vi "AlazarDSPGetModules.vi"(8 "error in (no error)":errorcluster, 11 "Handle":u32) -> (0 "error out":errorcluster, 1 "DSP Modules":u32[](array[numeric]), 2 "Return Code":u32, 3 "Handle":u32)   [LabVIEW 2018]
uses:
  ATSApi.dll
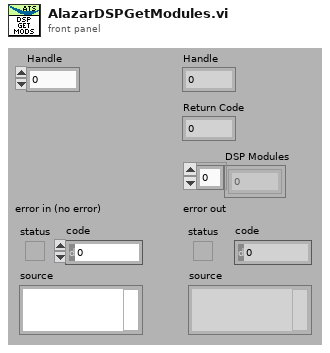
[diagram p1: front panel]
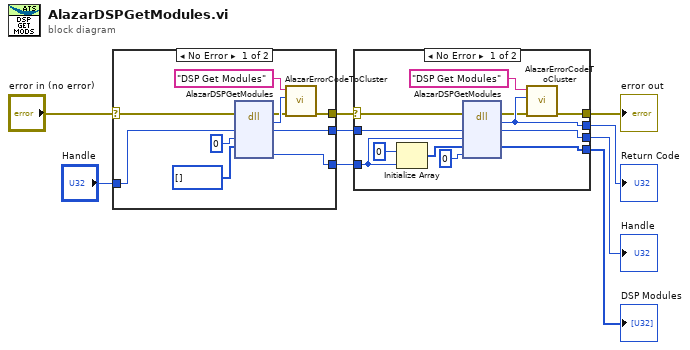
[diagram p0: block diagram]
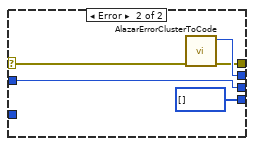
[diagram p2: hidden frame]
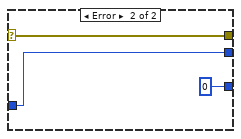
[diagram p3: hidden frame]
diagram:
  n1 = case shown="No Error" "error in (no error)" {
    selector: "error in (no error)" -> [w11 w22]
    tunnel: [w16 w22] -> w1
    tunnel: "Handle" -> [w19 w21]
    tunnel: [w15 w21] -> w6
    tunnel: [w13 0] -> w7
    frame No Error {
      n2 = dll-call lib="ATSApi.dll" fn="AlazarDSPGetModules"(error in=w11, "handle"=w19, "numEntries"=u32 0, "modules"=u32[] []) -> (error out=w10:errorcluster, "return type"=w18:u32, "handle"=w15:u32, "numModules"=w13:u32)  [unwired: 5 in, 1 out]
      n3 = call "AlazarErrorCodeToCluster.vi"("error in (no error)"=w10, "Error Code In"=w18, "Message"="DSP Get Modules") -> ("error out"=w16:errorcluster)  [unwired: 7 in, 1 out]
    }
    frame Error {
    }
  }
  n4 = case shown="No Error" w1 {
    selector: w1 -> [w24 w39]
    tunnel: [w31 w35] -> w4
    tunnel: [w33 w38] -> w5
    tunnel: w6 -> [w34 w37]
    tunnel: [w30 w37] -> w3
    tunnel: w7 -> [w29 _]
    tunnel: [w26 u32[] []] -> w2
    frame No Error {
      n5 = Initialize Array(u32 0, w29) -> (w27:u32[])
      n6 = dll-call lib="ATSApi.dll" fn="AlazarDSPGetModules"(error in=w24, "handle"=w34, "numEntries"=w29, "modules"=w27, "numModules"=u32 0) -> (error out=w23:errorcluster, "return type"=w33:u32, "handle"=w30:u32, "modules"=w26:u32[])  [unwired: 4 in, 1 out]
      n7 = call "AlazarErrorCodeToCluster.vi"("error in (no error)"=w23, "Error Code In"=w33, "Message"="DSP Get Modules") -> ("error out"=w31:errorcluster)  [unwired: 7 in, 1 out]
    }
    frame Error {
      n8 = call "AlazarErrorClusterToCode.vi"("error in (no error)"=w39) -> ("error out"=w35:errorcluster, "Error Code"=w38:u32)  [unwired: 9 in]
    }
  }
  "Handle" <- w3
  "error out" <- w4
  "Return Code" <- w5
  "DSP Modules" <- w2
